vi "_findLatestConnectionForPID.vi"(8 "error in (no error)":errorcluster, 10 "PID":i64, 11 "tWorkerController in":refnum<class "tWorkerController.lvclass">) -> (0 "error out":errorcluster, 1 "Found?":bool, 2 "Connections":T1, 3 "tWorkerController out":refnum<class "tWorkerController.lvclass">)   [LabVIEW 2013, in "tWorkerController.lvlib" / "tWorkerController.lvclass"]
uses:
  tWorkerController.lvclass
  _tcpConnection.ctl
  <vilib>/ActorFramework/Message Enqueuer/Message Enqueuer.lvclass
  tWorkerController.lvclass/tWorkerController.ctl
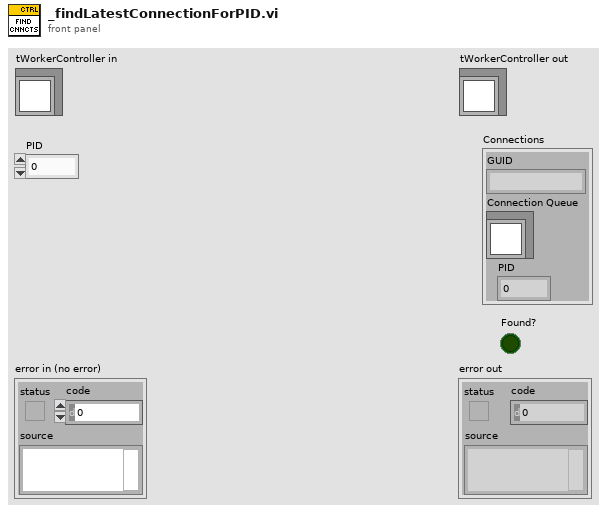
[diagram p1: front panel]
types:
  T1 = typedef "tWorkerController.lvlib/tWorkerController.lvclass/_tcpConnection.ctl" = cluster{"GUID":string, "Connection Queue":refnum<class "Message Enqueuer.lvclass">, "PID":i64}
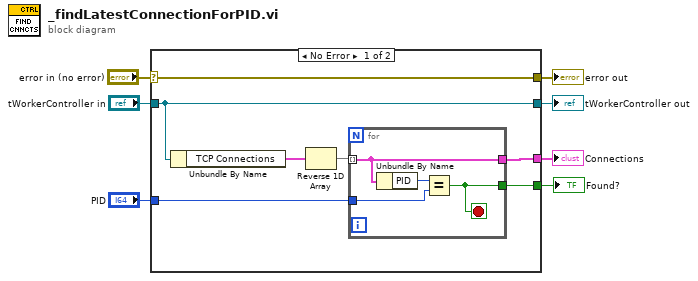
[diagram p0: block diagram]
diagram:
  n1 = case shown="No Error" "error in (no error)" {
    selector: "error in (no error)" -> [w14 w20]
    tunnel: [w14 w20] -> w6
    tunnel: [w13 w19] -> w4
    tunnel: "tWorkerController in" -> [w13 w19]
    tunnel: "PID" -> [w12 _]
    tunnel: [w11 _] -> w2
    tunnel: [w10 _] -> w1
    frame No Error {
      n2 = Unbundle By Name(w13) -> ("TCP Connections"=w8:T1[])
      n3 = Reverse 1D Array(array=w8) -> (reversed array=w9:T1[])
      n4 = for {
        tunnel: w9 -> [w16] mode=indexing
        tunnel: w12 -> [w17]
        tunnel: [w16] -> w10
        tunnel: [w15] -> w11
        stop <- w15 stop-if-true
        n5 = Unbundle By Name(w16) -> ("PID"=w18:i64)
        n6 = Equal?(x=w18, y=w17) -> (x = y?=w15:bool)
      }
    }
    frame Error {
    }
  }
  "error out" <- w6
  "tWorkerController out" <- w4
  "Connections" <- w1
  "Found?" <- w2
